vi "Do.vi"(8 "error in (no error)":errorcluster, 10 "Actor in":refnum<class "Actor.lvclass">, 11 "Read Packet Msg":refnum<class "Read Packet Msg.lvclass">) -> (0 "error out":errorcluster, 2 "Actor out":refnum<class "Actor.lvclass">)   [LabVIEW 2015, in "SCADA Communcations Actor.lvlib" / "Read Packet Msg.lvclass"]
doc: "(<B>Filename</B>: Actor Framework.lvlib:Message.lvclass:Do.vi)\n\nDefines what a message does when it is received by an actor. Generally, a message instructs an actor to invoke one of its methods. By default, this method does nothing. A child class must override it to define behavior. Create a child class by using the Actor Framework Message Maker dialog box."
uses:
  Read Packet Msg.lvclass
  <vilib>/ActorFramework/Actor/Actor.lvclass
  SCADA Communications/SCADA Communications.lvclass
  TCPIP Communications Framework/TCPIP Communications Messages/Packet Msg/Packet Msg.lvclass
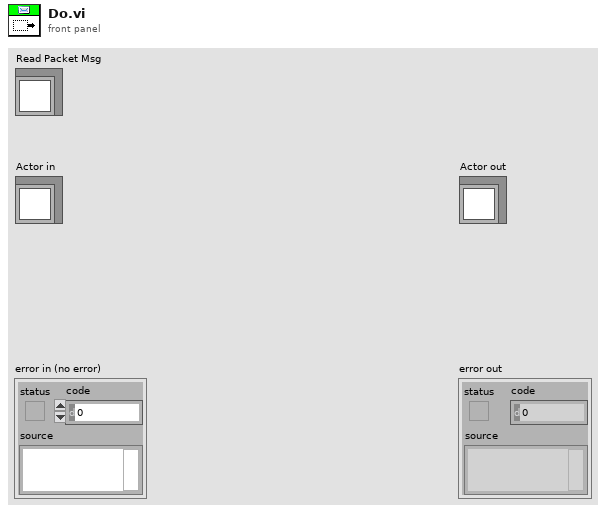
[diagram p1: front panel]
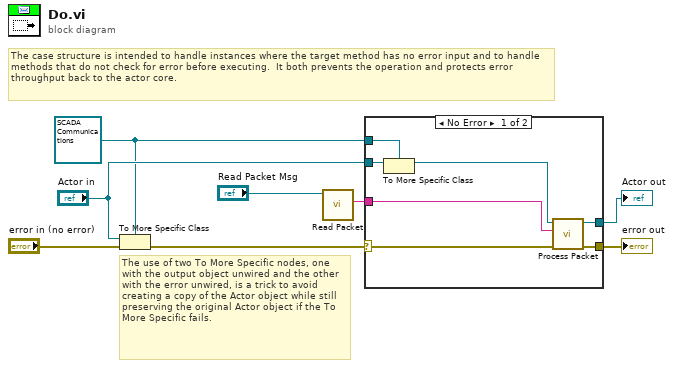
[diagram p0: block diagram]
diagram:
  w1 = refnum<class "SCADA Communications.lvclass"> refnum ("SCADA Communcations Actor.lvlib:SCADA Communications.lvclass")
  # "The use of two To More Specific nodes, one with the output object unwired and the other with the error unwired, is a trick to avoid creating a copy of the Actor object while still preserving the original Actor object if the To More Specific fails."
  # "The case structure is intended to handle instances where the target method has no error input and to handle methods that do not check for error before executing.  It both prevents the operation and protects error throughput back to the actor core."
  n1 = To More Specific Class(target class=w1, reference="Actor in", error in="error in (no error)") -> (error out=w7:errorcluster)  [unwired: 1 out]
  n2 = call "Read Packet.vi"("Packet Msg in"="Read Packet Msg") -> ("Packet"=w6:string)  [unwired: 9 in, 1 out]
  n3 = case shown="No Error" w7 {
    selector: w7 -> [w13 w17]
    tunnel: [w12 w17] -> w3
    tunnel: [w11 w16] -> w4
    tunnel: "Actor in" -> [w15 w16]
    tunnel: w1 -> [w14 _]
    tunnel: w6 -> [w9 _]
    frame No Error {
      n4 = To More Specific Class(target class=w14, reference=w15) -> (specific class reference=w10:refnum<class "SCADA Communications.lvclass">)  [unwired: 1 in, 1 out]
      n5 = call "Process Packet.vi"("error in (no error)"=w13, "Packet"=w9, "SCADA Communications in"=w10) -> ("error out"=w12:errorcluster, "SCADA Communications out"=w11:refnum<class "SCADA Communications.lvclass">)  [unwired: 7 in]
    }
    frame Error {
      # "If type check fails, pass the original object out again."
    }
  }
  "error out" <- w3
  "Actor out" <- w4
